vi "TEC-Convert-Bytes.vi"(11 "Frames Read":u8[](array[numeric])) -> (0 "Short-Circuited to Vcc ?":bool, 1 "Open TC ?":bool, 2 "CJC Temp [°C]":dbl, 3 "TEC Temp [°C]":dbl, 4 "Short-Circuited to GND ?":bool, 5 "General Error Alert":bool)   [LabVIEW 2018]
panel:
  out "16bit integer 2":i16
  out "16bit integer":i16
  out "Boolean array 4":bool[](array[boolean])
  out "Boolean array 3":bool[](array[boolean])
  out "Boolean array 2":bool[](array[boolean])
  out "Boolean array":bool[](array[boolean])
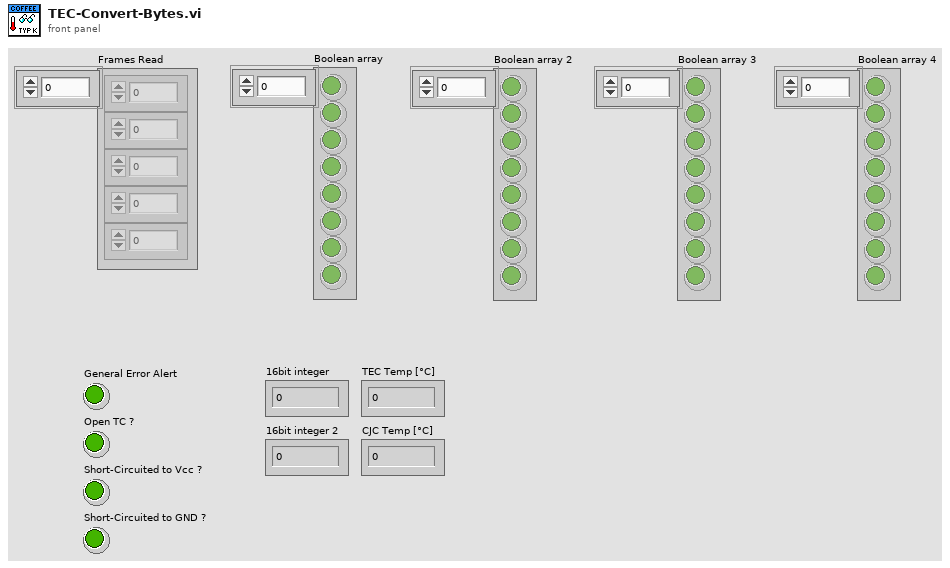
[diagram p1: front panel]
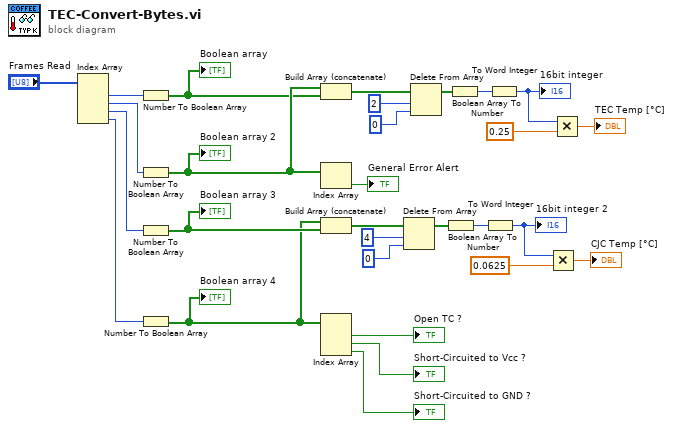
[diagram p0: block diagram]
diagram:
  n1 = Index Array "Index Array"(array="Frames Read") -> (element #1=w21:u8, element #2=w22:u8, element #3=w28:u8, element #4=w29:u8)  [unwired: 4 in]
  n2 = Number To Boolean Array(number=w21) -> (Boolean array=w19:bool[])
  "Boolean array" <- w19
  n3 = Number To Boolean Array(number=w22) -> (Boolean array=w20:bool[])
  "Boolean array 2" <- w20
  n4 = Number To Boolean Array(number=w28) -> (Boolean array=w2:bool[])
  "Boolean array 3" <- w2
  n5 = Number To Boolean Array(number=w29) -> (Boolean array=w1:bool[])
  "Boolean array 4" <- w1
  n6 = Build Array (concatenate)(w20, w19) -> (w18:bool[])
  n7 = Index Array(array=w20) -> (element=→"General Error Alert":bool)  [unwired: 1 in]
  n8 = Build Array (concatenate)(w1, w2) -> (w3:bool[])
  n9 = Index Array(array=w1) -> (element #1=→"Open TC ?":bool, element #2=→"Short-Circuited to Vcc ?":bool, element #3=→"Short-Circuited to GND ?":bool)  [unwired: 3 in]
  n10 = Delete From Array(array=w3, length=4, index=0) -> (array with subset deleted=w6:bool[])  [unwired: 1 out]
  n11 = Delete From Array(array=w18, length=2, index=0) -> (array with subset deleted=w15:bool[])  [unwired: 1 out]
  n12 = Boolean Array To Number(Boolean array=w6) -> (number=w7:u32)
  n13 = Boolean Array To Number(Boolean array=w15) -> (number=w14:u32)
  n14 = To Word Integer(number=w7) -> (16bit integer=w8:i16)
  "16bit integer 2" <- w8
  n15 = To Word Integer(number=w14) -> (16bit integer=w13:i16)
  "16bit integer" <- w13
  n16 = Multiply(x=w8, y=0.0625) -> (x*y=→"CJC Temp [°C]":dbl)
  n17 = Multiply(x=w13, y=0.25) -> (x*y=→"TEC Temp [°C]":dbl)
